vi "编辑配方.vi"() -> ()   [LabVIEW 2018]
panel:
  out "所在行号":string="所在行号"
  out "档位名称":string="档位名称"
  out "序号":string="序号"
  out "子配方":string="子配方"
  out "子配方":string[][](array[string])
  out "档位终止行号":string="档位终止行号"
  out "档位起始行号":string="档位起始行号"
  in  "退出":bool
  in  "确定写入":bool
  out "说明":string="说明"
  out "详细位置":string="详细位置"
  out "配方编号":string="配方编号"
  in  "编辑配方":string[][](array[string])
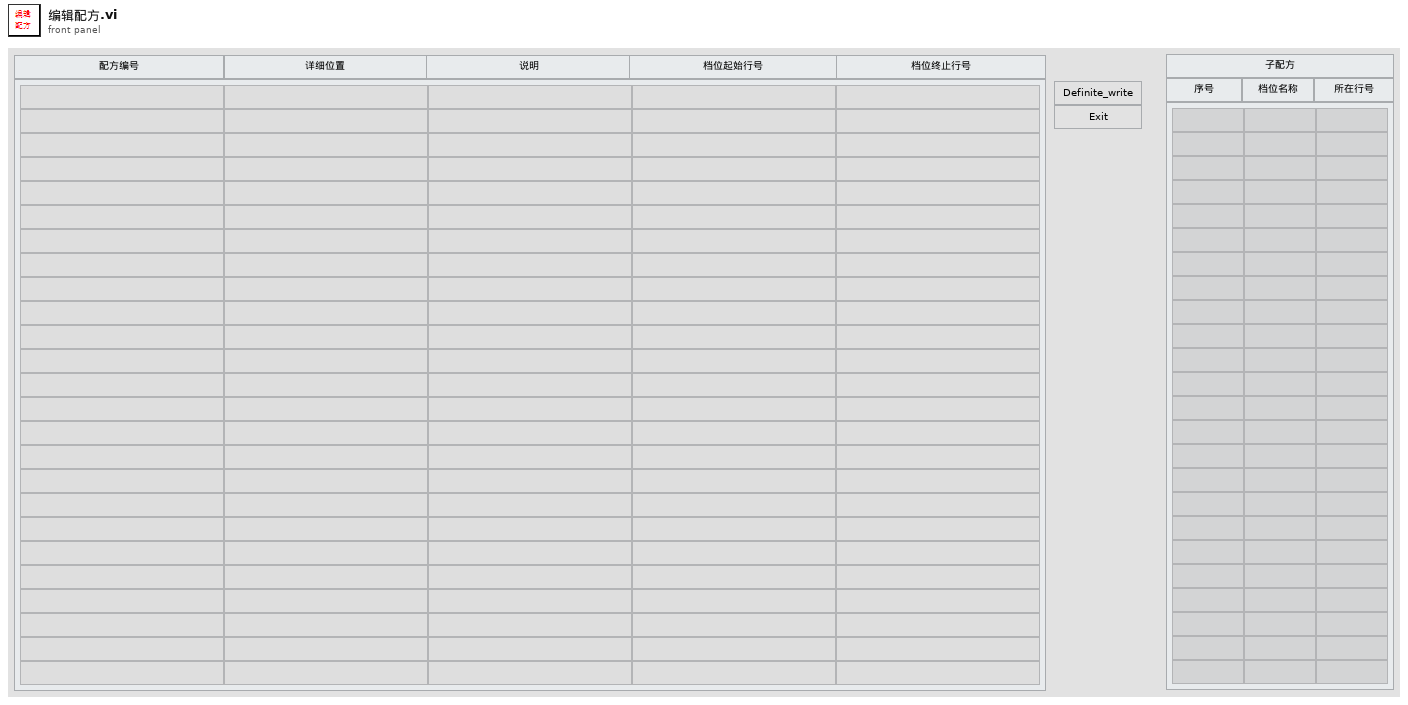
[diagram p1: front panel]
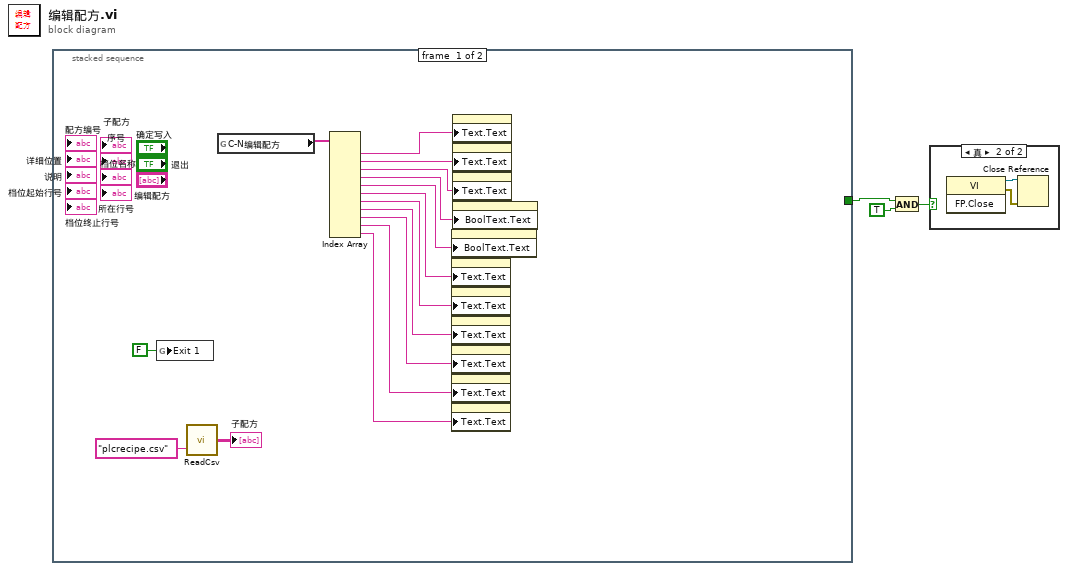
[diagram p0: block diagram]
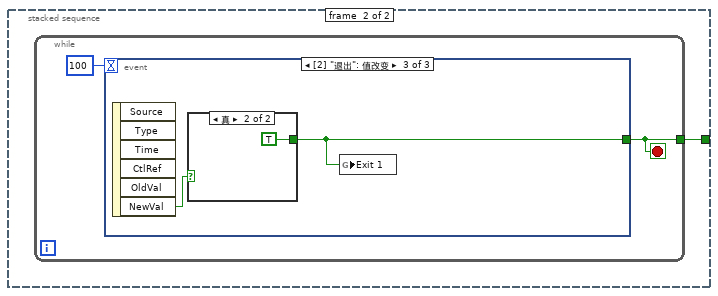
[diagram p2: hidden frame]
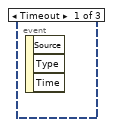
[diagram p3: hidden frame]
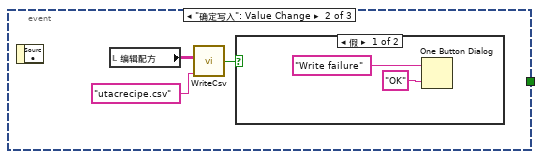
[diagram p4: hidden frame]
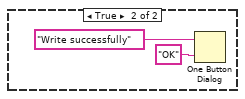
[diagram p5: hidden frame]
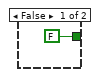
[diagram p6: hidden frame]
diagram:
  n1 = stacked-sequence {
    tunnel: [_ w19] -> w1
    frame #0 {
      n2 = global write "全局 1.vi" "Exit 1"(FALSE ("Exit 1")) -> ()
      n3 = call "ReadCsv.vi"("相对路径"="plcrecipe.csv") -> ("all rows"=→"子配方":string[][])  [unwired: 1 in]
      n4 = global read "全局 1.vi" "C-N编辑配方"() -> (w18:string[])
      n5 = Index Array(array=w18) -> (element #1=w17:string, element #2=w16:string, element #3=w15:string, element #4=w14:string, element #5=w13:string, element #6=w9:string, element #7=w8:string, element #8=w7:string, element #9=w6:string, element #10=w5:string, element #11=w4:string)  [unwired: 11 in]
      n6 = property on="退出" class="Bool"("BoolText.Text"=w13) -> ()  [unwired: 2 in, 2 out]
      n7 = property on="档位起始行号" class="Str"("Text.Text"=w9) -> ()  [unwired: 2 in, 2 out]
      n8 = property on="档位终止行号" class="Str"("Text.Text"=w8) -> ()  [unwired: 2 in, 2 out]
      n9 = property on="子配方" class="Str"("Text.Text"=w7) -> ()  [unwired: 2 in, 2 out]
      n10 = property on="序号" class="Str"("Text.Text"=w6) -> ()  [unwired: 2 in, 2 out]
      n11 = property on="档位名称" class="Str"("Text.Text"=w5) -> ()  [unwired: 2 in, 2 out]
      n12 = property on="所在行号" class="Str"("Text.Text"=w4) -> ()  [unwired: 2 in, 2 out]
      n13 = property on="配方编号" class="Str"("Text.Text"=w17) -> ()  [unwired: 2 in, 2 out]
      n14 = property on="详细位置" class="Str"("Text.Text"=w16) -> ()  [unwired: 2 in, 2 out]
      n15 = property on="说明" class="Str"("Text.Text"=w15) -> ()  [unwired: 2 in, 2 out]
      n16 = property on="确定写入" class="Bool"("BoolText.Text"=w14) -> ()  [unwired: 2 in, 2 out]
    }
    frame #1 {
      n17 = while {
        tunnel: [w20] -> w19
        stop <- w20 stop-if-true
        n18 = event shown="[2] \"退出\": 值改变" {
          selector: _ -> [_ _ _]
          dyn-events: _ -> [_ _ _]
          timeout: 100 -> [_ _ _]
          tunnel: [_ _ w29] -> w20
          event Timeout {
            n19 = event-data() -> ()  [unwired: 1 in, 3 out]
          }
          event "确定写入": Value Change {
            n20 = event-data() -> ()  [unwired: 1 in, 1 out]
            n21 = local read "编辑配方"() -> (w23:string[][])
            n22 = call "WriteCsv.vi"("相对路径"="utacrecipe.csv", "2D data"=w23) -> ("布尔"=w22:bool)  [unwired: 2 in]
            n23 = case shown="假" w22 {
              frame False {
                n24 = One Button Dialog(message="Write failure" ("消息"), button name ("OK")="OK" ("按钮名称（“确定”）")) -> ()  [unwired: 1 out]
              }
              frame True {
                n25 = One Button Dialog(message="Write successfully" ("消息"), button name ("OK")="OK" ("按钮名称（“确定”）")) -> ()  [unwired: 1 out]
              }
            }
          }
          event "退出": Value Change {
            n26 = event-data() -> ("NewVal"=w30:bool)  [unwired: 1 in, 5 out]
            n27 = case shown="真" w30 {
              tunnel: [FALSE TRUE] -> w29
              frame False {
              }
              frame True {
              }
            }
            n28 = global write "全局 1.vi" "Exit 1"(w29) -> ()
          }
        }
      }
    }
  }
  n29 = And(x=w1, y=TRUE) -> (x .and. y?=w2:bool)
  n30 = case shown="真" w2 {
    frame False {
    }
    frame True {
      n31 = invoke class="VI" method="FP.Close"() -> (reference out=w34:refnum<vi>, error out=w33:errorcluster)  [unwired: 3 in, 1 out]
      n32 = Close Reference(reference=w34, error in (no error)=w33) -> ()  [unwired: 1 out]
    }
  }
